vi "_Read.vi"(8 "error in (no error)":errorcluster, 10 "Count":i32, 11 "TCPStreamProxy in":refnum<class "TCPStream.lvclass">) -> (0 "error out":errorcluster, 2 "Data":string, 3 "TCPStreamProxy out":refnum<class "TCPStream.lvclass">)   [LabVIEW 2020, in "HTTP Utils.lvlib" / "TCPStream.lvclass"]
uses:
  TCPStream.lvclass
  TCPStream.lvclass/TCPStream.ctl
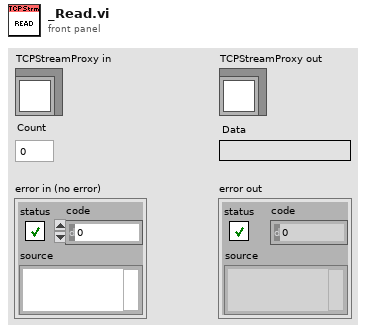
[diagram p1: front panel]
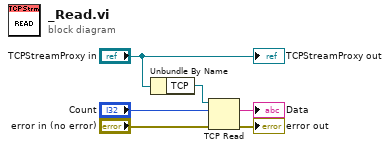
[diagram p0: block diagram]
diagram:
  n1 = Unbundle By Name("TCPStreamProxy in") -> ("TCP"=w5:refnum<k5>)
  n2 = TCP Read(connection ID=w5, bytes to read="Count", error in (no error)="error in (no error)") -> (data out=→"Data":string, error out=→"error out":errorcluster)  [unwired: 2 in, 1 out]
  "TCPStreamProxy out" <- "TCPStreamProxy in"
